vi "Validate RT Address.vi"(4 "RT Address (0-30)":u8, 6 "RT 1?":bool, 8 "error in (no error)":errorcluster, 11 "RT Config in":refnum<class "RT Config.lvclass">) -> (0 "error out":errorcluster, 3 "RT Config out":refnum<class "RT Config.lvclass">)   [LabVIEW 2016, in "RT Config.lvclass"]
uses:
  RT Config.lvclass
  PPLs/FPGA Interface.lvlibp/FPGA Interface/FPGA Interface.lvclass
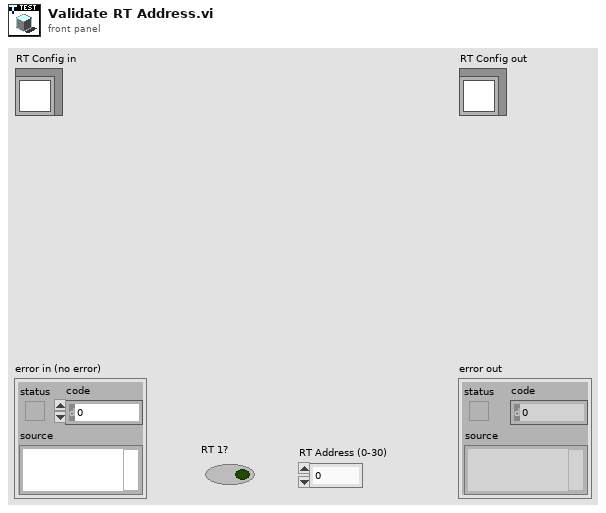
[diagram p1: front panel]
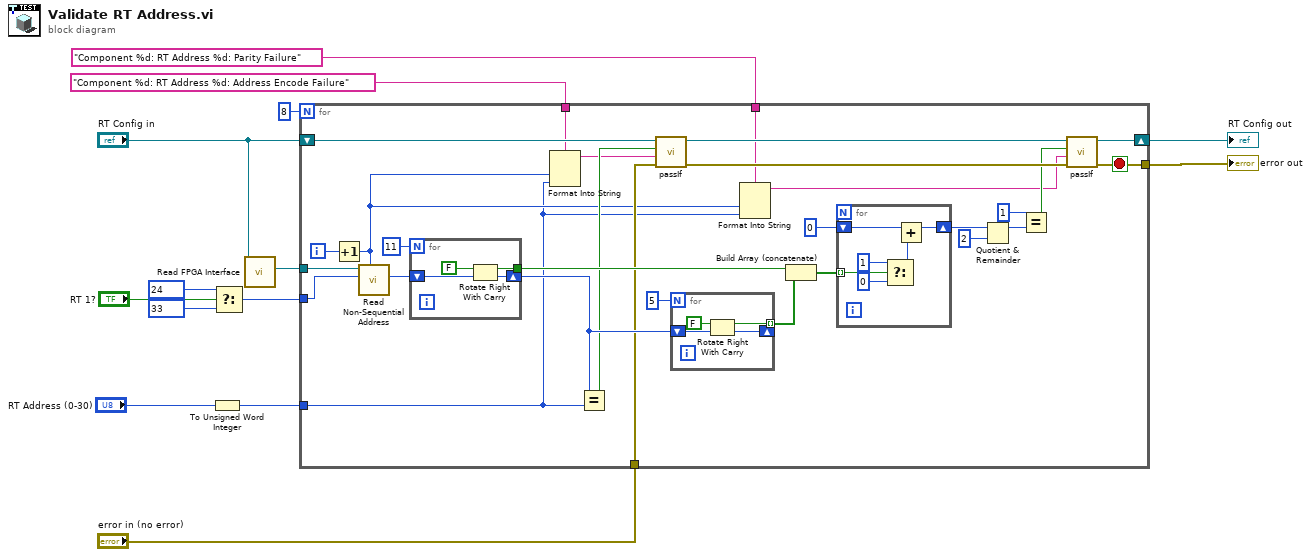
[diagram p0: block diagram]
diagram:
  n1 = To Unsigned Word Integer(number="RT Address (0-30)") -> (unsigned 16bit integer=w6:u16)
  n2 = Select(t=u16 24, s="RT 1?", f=u16 33) -> (s? t:f=w7:u16)
  n3 = call-dynamic "Read FPGA Interface.vi"("1553 Test in"="RT Config in") -> ("FPGA Interface"=w10:refnum<class "FPGA Interface.lvclass">)  [unwired: 8 in, 2 out]
  n4 = for {
    N: 8 -> [_]
    tunnel: w10 -> [w43]
    shift-right: [w27] -> w8
    shift-left: "RT Config in" -> [w28]
    tunnel: w7 -> [w42]
    tunnel: w6 -> [w18]
    tunnel: [w24] -> w5
    tunnel: "error in (no error)" -> [w22]
    tunnel: "Component %d: RT Address %d: Address Encode Failure" -> [w20]
    tunnel: "Component %d: RT Address %d: Parity Failure" -> [w21]
    i -> [w41]
    stop <- w24 stop-if-true
    n5 = Increment(x=w41) -> (x+1=w19:i32)
    n6 = call-dynamic "Read Non-Sequential Address.vi"("Target IC (1-8)"=w19, "Address"=w42, "FPGA Interface in"=w43) -> ("Data"=w40:u16)  [unwired: 7 in, 1 out]
    n7 = for {
      N: 11 -> [_]
      tunnel: [w56] -> w36
      shift-right: [w55] -> w37
      shift-left: w40 -> [w57]
      n8 = Rotate Right With Carry(2:w57, 3:FALSE ("carry")) -> (0:w55:u16, 1:w56:bool)
    }
    n9 = Format Into String(format string=w20, w19, w18) -> (resulting string=w17:string)  [unwired: 2 in, 1 out]
    n10 = Equal?(x=w37, y=w18) -> (x = y?=w26:bool)
    n11 = call-dynamic "passIf.vi"("error in (no error)"=w22, "message (\"\")"=w17, "pass"=w26, "TestCase in"=w28) -> ("error out"=w25:errorcluster, "TestCase out"=w29:refnum<class "RT Config.lvclass">)  [unwired: 6 in]
    n12 = for {
      N: 5 -> [_]
      shift-right: [w52] -> _
      shift-left: w37 -> [w53]
      tunnel: [w51] -> w35 mode=indexing
      n13 = Rotate Right With Carry(2:w53, 3:FALSE ("carry")) -> (0:w52:u16, 1:w51:bool)
    }
    n14 = Format Into String(format string=w21, w19, w18) -> (resulting string=w16:string)  [unwired: 2 in, 1 out]
    n15 = Build Array (concatenate)(w36, w35) -> (w34:bool[])
    n16 = for {
      tunnel: w34 -> [w47] mode=indexing
      shift-right: [w48] -> w32
      shift-left: 0 -> [w49]
      n17 = Select(t=1, s=w47, f=0) -> (s? t:f=w44:i32)
      n18 = Add(x=w49, y=w44) -> (x+y=w48:i32)
    }
    n19 = Quotient & Remainder(x=w32, y=2) -> (x-y*floor(x/y)=w30:i32)  [unwired: 1 out]
    n20 = Equal?(x=1, y=w30) -> (x = y?=w23:bool)
    n21 = call-dynamic "passIf.vi"("error in (no error)"=w25, "message (\"\")"=w16, "pass"=w23, "TestCase in"=w29) -> ("error out"=w24:errorcluster, "TestCase out"=w27:refnum<class "RT Config.lvclass">)  [unwired: 6 in]
  }
  "error out" <- w5
  "RT Config out" <- w8
